vi "setReset.vi"(8 "error in":errorcluster, 10 "axis in":u8, 11 "connection ID":refnum<k5>) -> (0 "error out":errorcluster, 2 "axis out":u8, 3 "connection ID":refnum<k5>)   [LabVIEW 2019]
panel:
  in  "Set Command":string="com.attocube.amc.control.setReset"
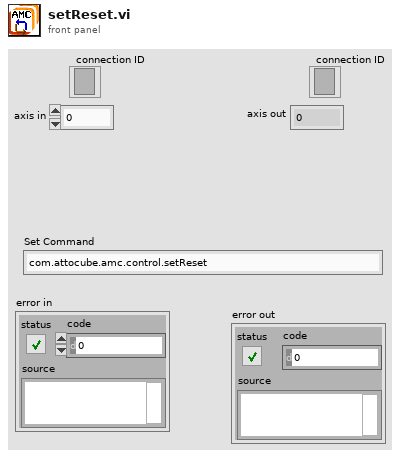
[diagram p1: front panel]
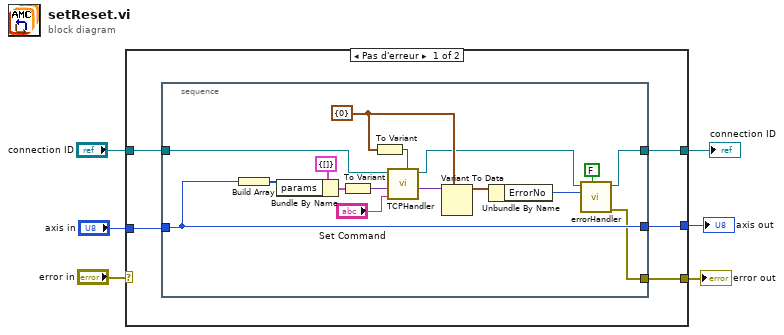
[diagram p0: block diagram]
diagram:
  n1 = case shown="Pas d'erreur" "error in" {
    selector: "error in" -> [_ w30]
    tunnel: "axis in" -> [w11 w29]
    tunnel: [w7 w30] -> w5
    tunnel: [w8 w29] -> w4
    tunnel: [w9 w28] -> w3
    tunnel: "connection ID" -> [w10 w28]
    frame No Error {
      n2 = stacked-sequence {
        tunnel: [w12] -> w9
        tunnel: w10 -> [w17]
        tunnel: w11 -> [w19]
        tunnel: [w19] -> w8
        tunnel: [w18] -> w7
        frame #0 {
          w15 = cluster{"ErrorNo":i32} {"ErrorNo"=0} ("input cluster")
          n3 = Build Array(w19) -> (w23:u8[])
          n4 = Bundle By Name(cluster=cluster{"params":i32[]} {"params"=[]} ("input cluster"), "params"=w23) -> (w24:cluster{"params":i32[]})
          n5 = To Variant(anything=w24) -> (Variant=w25:variant)
          n6 = To Variant(anything=w15) -> (Variant=w16:variant)
          n7 = call <userlib>:"TCPHandler.vi"("result Types"=w16, "method"="Set Command", "params"=w25, "connection ID"=w17) -> ("result"=w21:variant, "connection ID"=w13:refnum<k5>)  [unwired: 5 in, 1 out]
          n8 = Variant To Data(type=w15, Variant=w21) -> (data=w26:cluster{"ErrorNo":i32})  [unwired: 1 in, 1 out]
          n9 = Unbundle By Name(w26) -> ("ErrorNo"=w27:i32)
          n10 = call <userlib>:"errorHandler.vi"("show popup"=FALSE, "error number"=w27, "connection ID"=w13) -> ("error out"=w18:errorcluster, "connection ID"=w12:refnum<k5>)  [unwired: 7 in]
        }
      }
    }
    frame Error {
    }
  }
  "error out" <- w5
  "axis out" <- w4
  "connection ID" <- w3
